vi "CameraControl.vi"() -> ()   [LabVIEW 2013]
uses:
  QImaging_Basic/Controls/Parameter.ctl
panel:
  out "abort err":errorcluster
  in  "Abort":bool
  in  "Trig":bool
  out "Intensity Graph":u16[][](graph)
  out "CCD Height":u32=1 min=1 max=4 step=1
  out "CCD Width":u32=1 min=1 max=4 step=1
  in  "Binning":u32=1 min=1 max=4 step=1
  out "Open Cam Error":i32
  out "LibCam Error":u32
  out "LibOpen error":i32
  in  "Stop Camera":bool
  in  "Start Camera":bool
  in  "Exposure Time":u32
  out "ParamVal":u32[](array[numeric])
  out "Camera Id":u32
  out "error out":errorcluster
  in  "error in (no error)":errorcluster
  in  "Stop":bool
  # "Hardware"
  # "Freerun"
  # "Image Width"
  # "Image Height"
  # "Image Size"
  # "CCD Type"
  # "CCD Width"
  # "CCD Height"
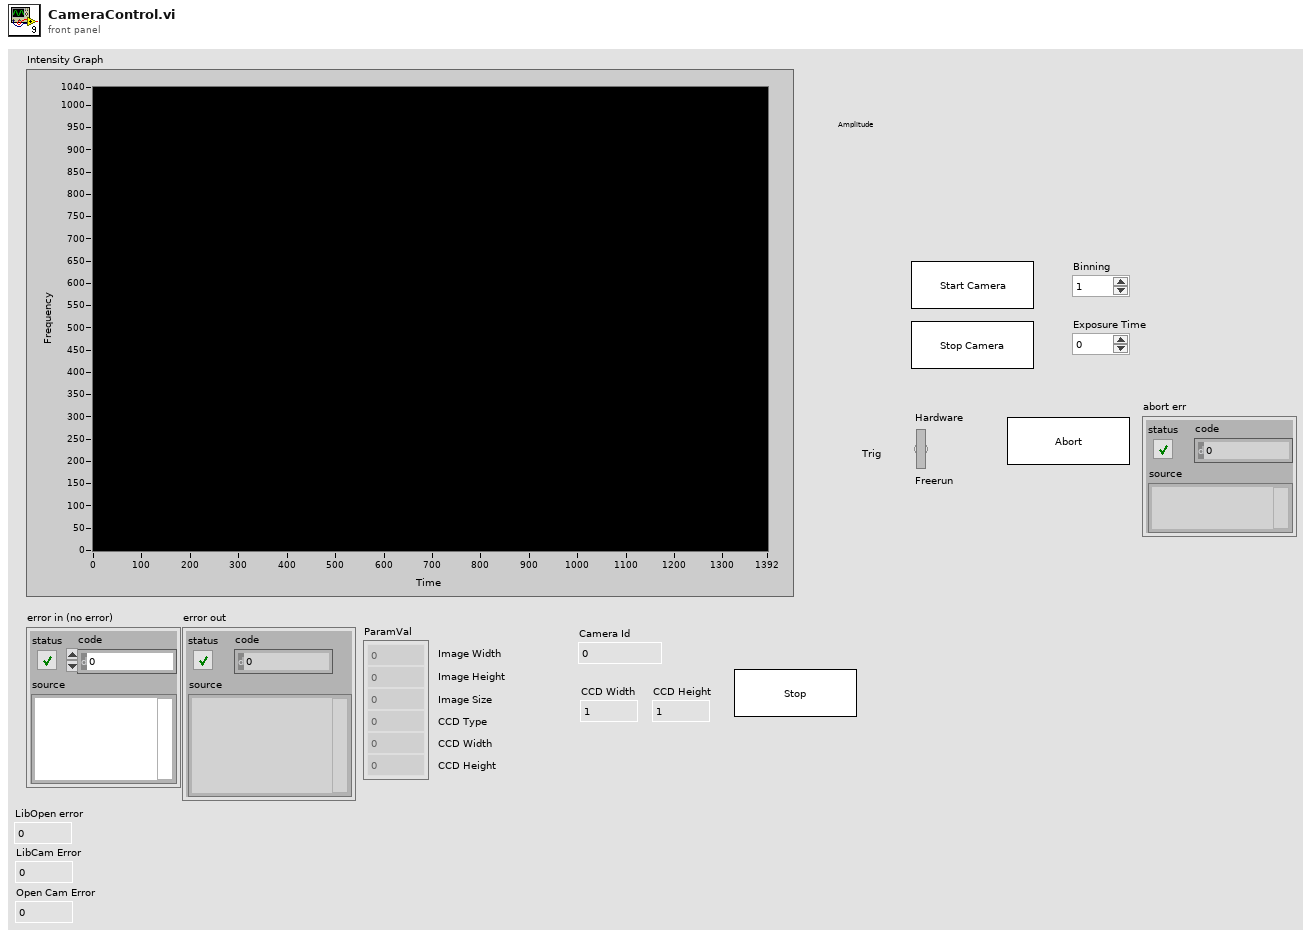
[diagram p1: front panel]
types:
  T1 = typedef "Parameter.ctl" = enum32{"Gain ", "Offset", "Exposure", "Binning", "HzBinning", "VtBinning", "Readout speed", "Trigger Type", "Color Wheel", "Cooler Active", "Exposure red", "Exposure blue", "Image format", "ROI X", "ROI Y", "ROI Width", "ROI Height"}
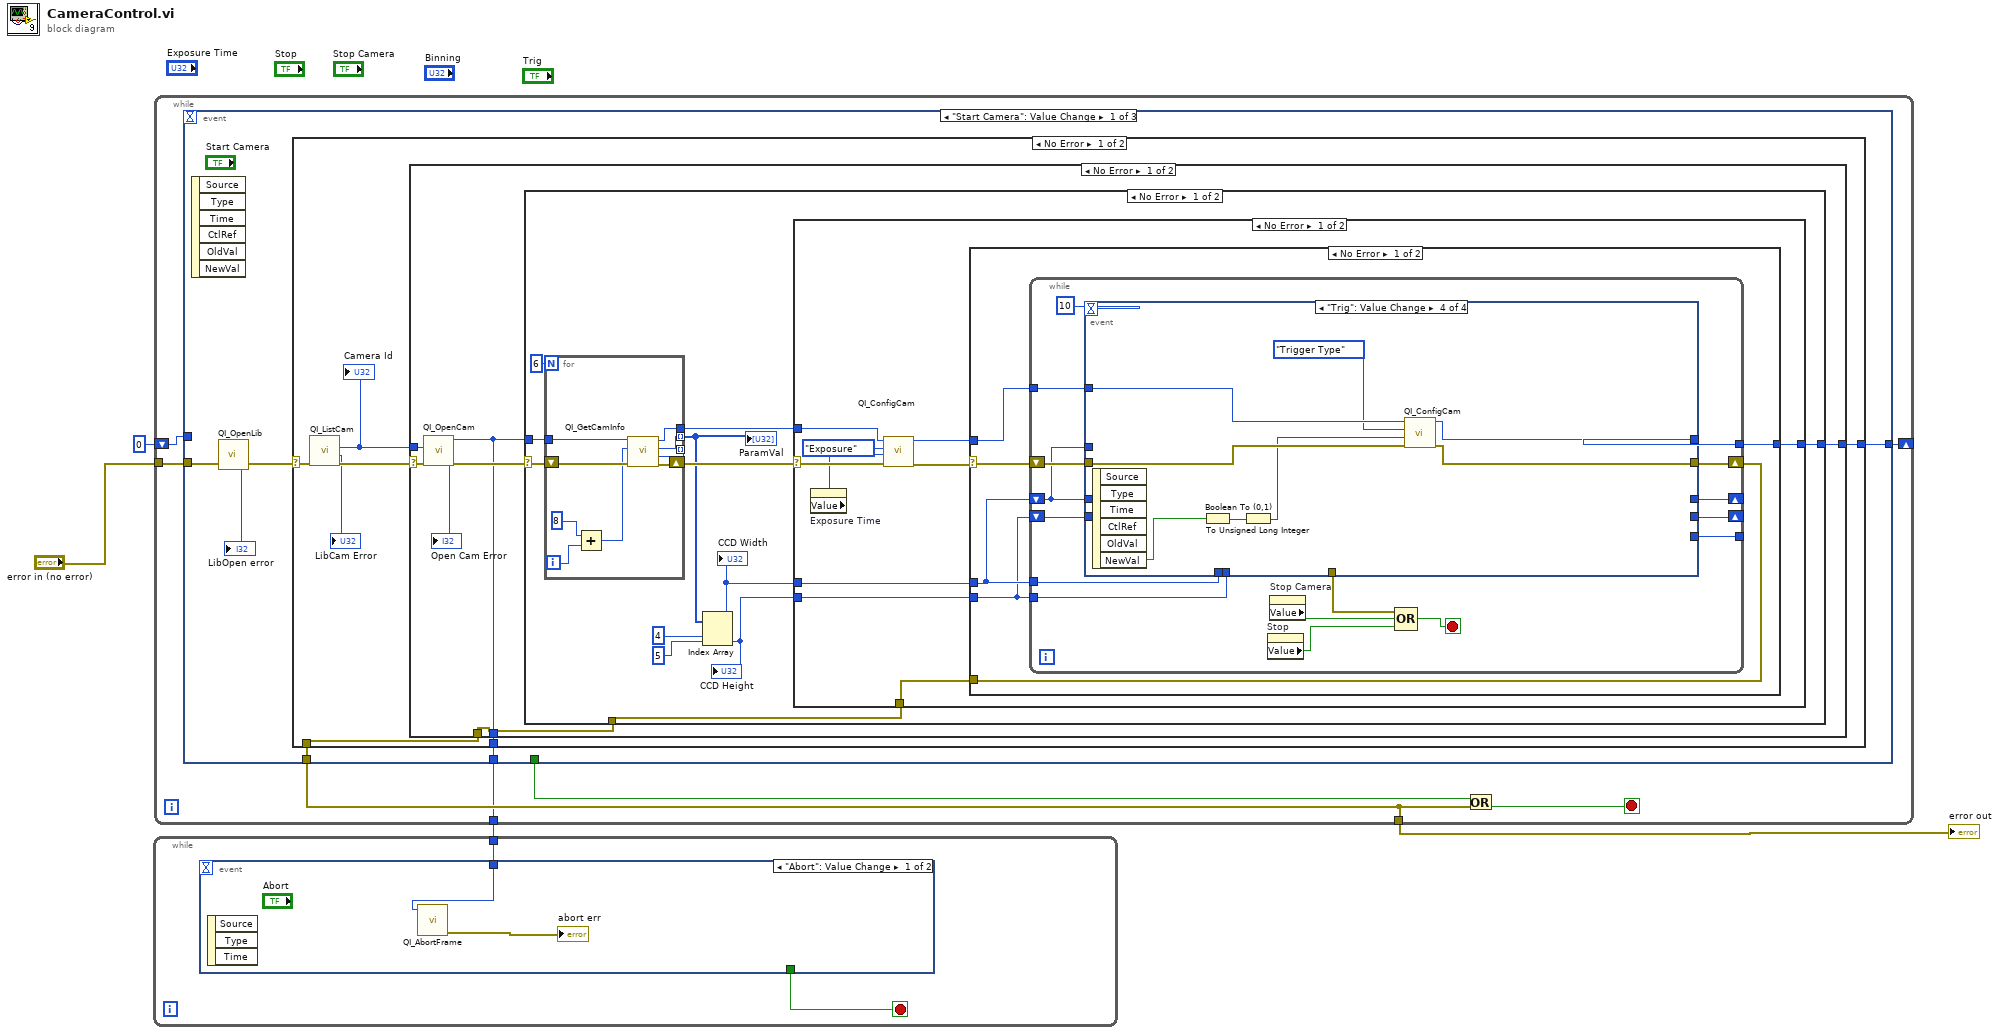
[diagram p0: block diagram]
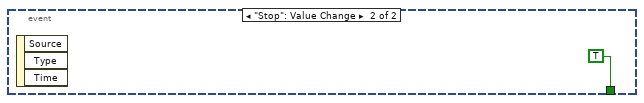
[diagram p2: hidden frame]
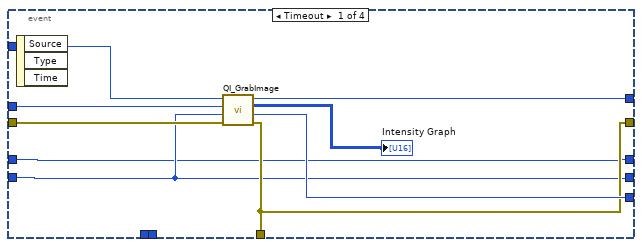
[diagram p3: hidden frame]
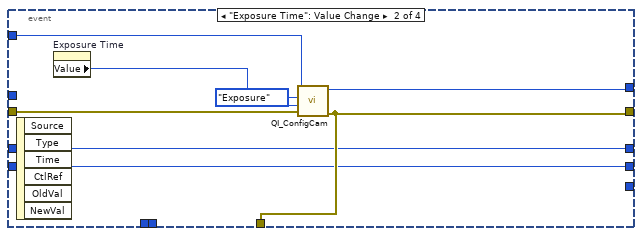
[diagram p4: hidden frame]
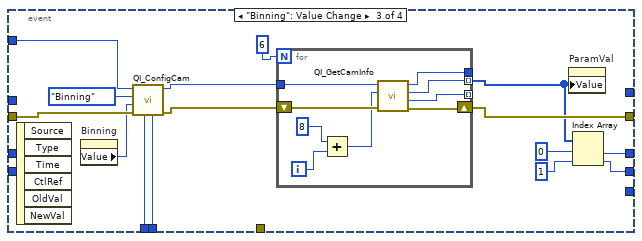
[diagram p5: hidden frame]
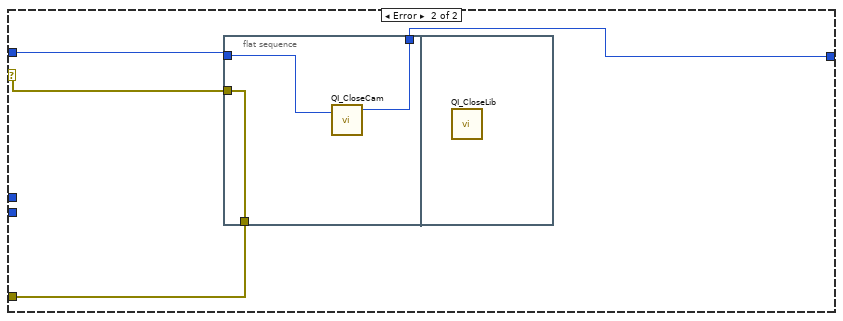
[diagram p6: hidden frame]
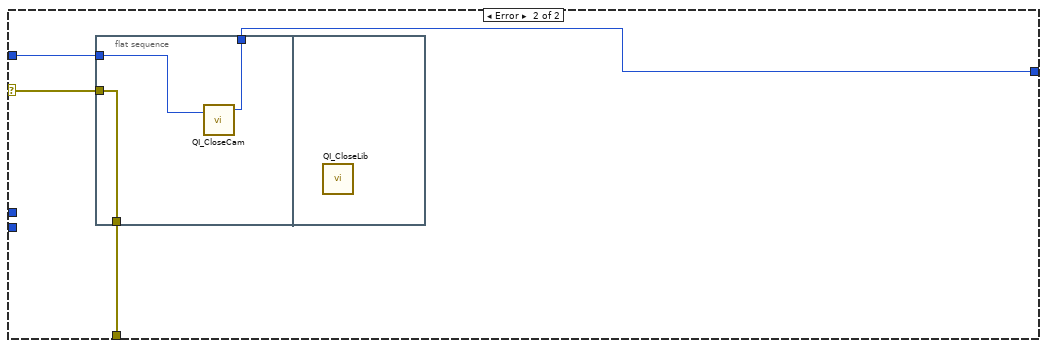
[diagram p7: hidden frame]
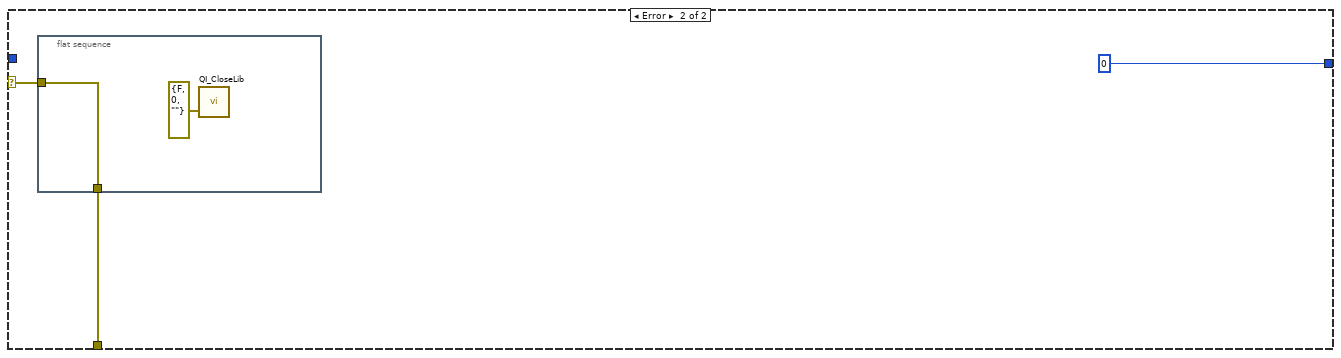
[diagram p8: hidden frame]
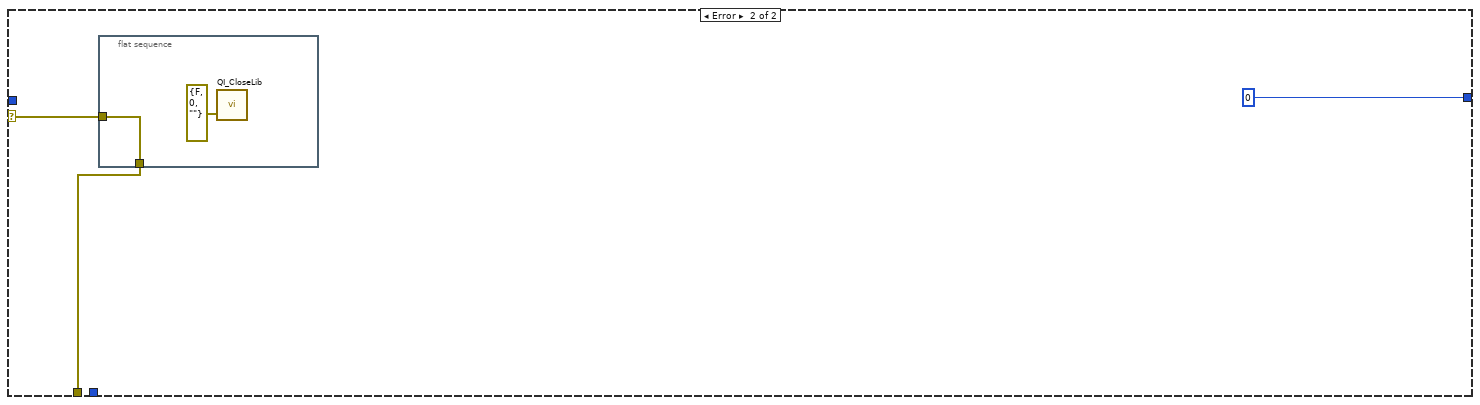
[diagram p9: hidden frame]
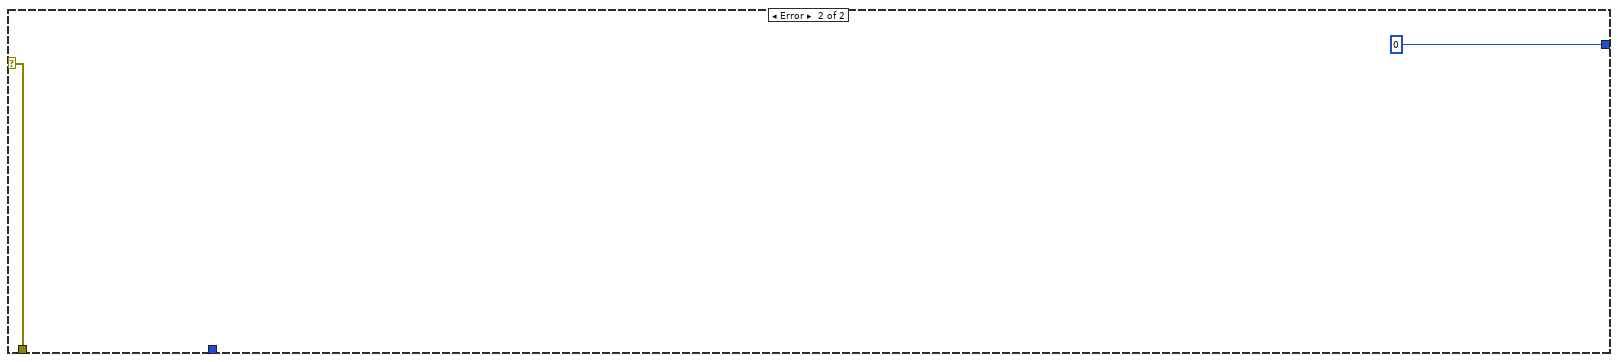
[diagram p10: hidden frame]
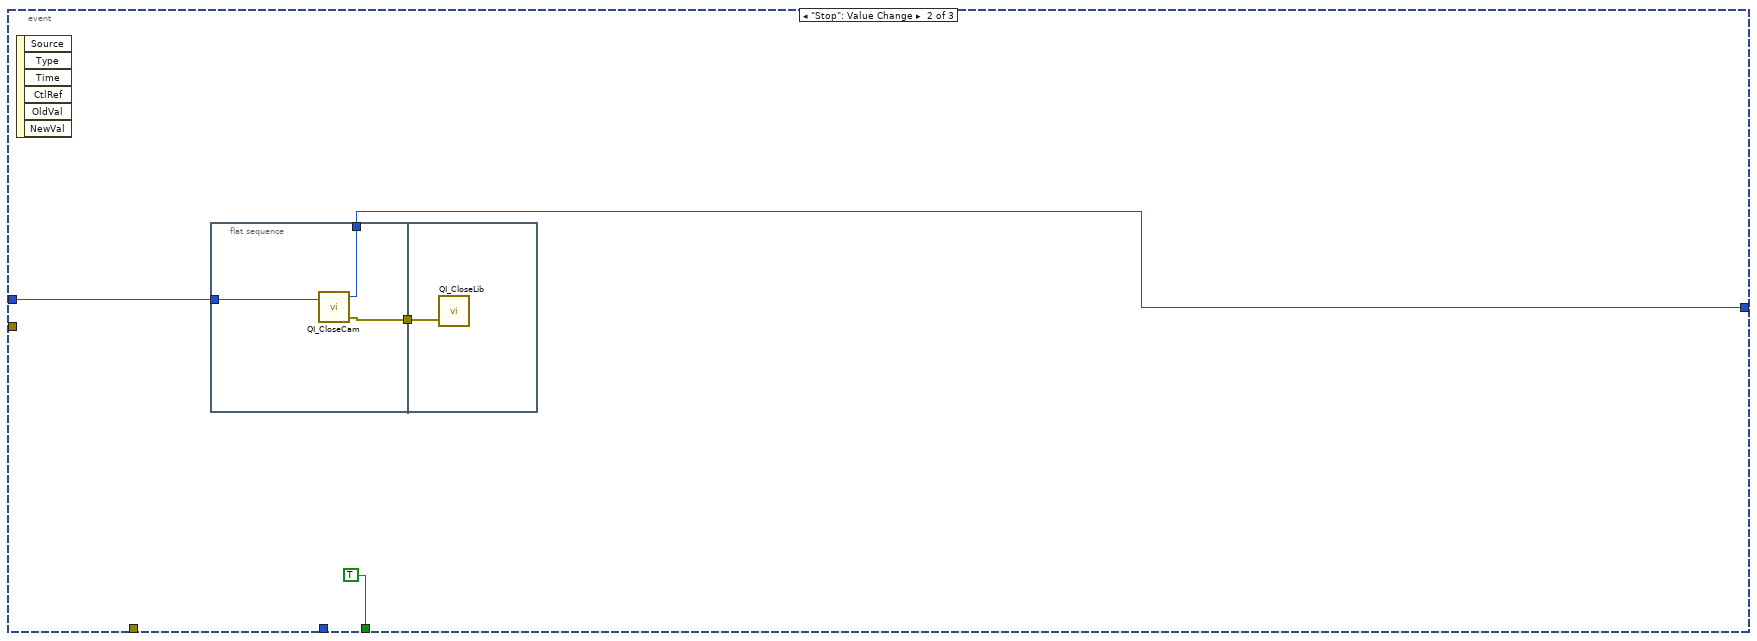
[diagram p11: hidden frame]
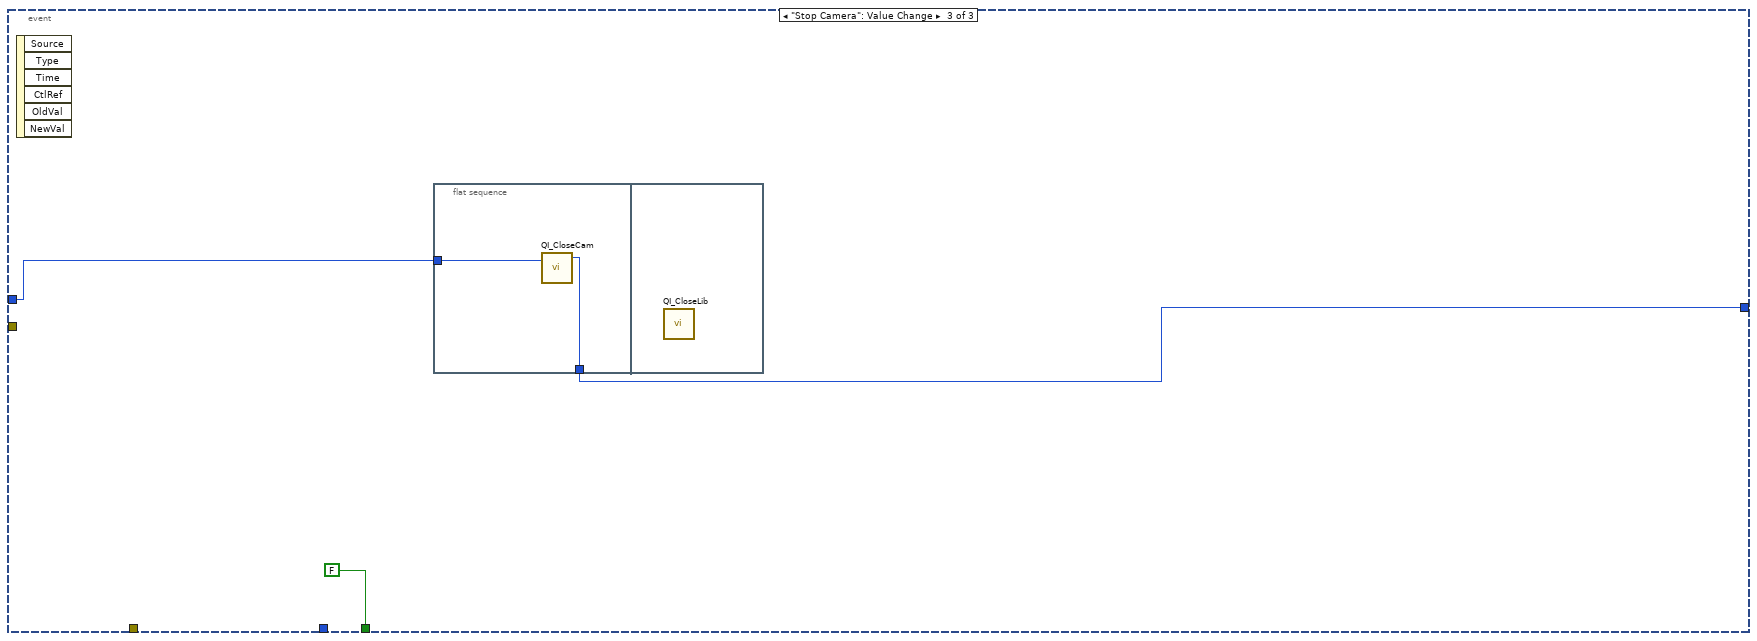
[diagram p12: hidden frame]
diagram:
  n1 = while {
    tunnel: "error in (no error)" -> [w11]
    shift-right: [w9] -> _
    shift-left: u32 0 ("Camera Handle") -> [w8]
    tunnel: [w7] -> w2
    tunnel: [w5] -> w1
    stop <- w6 stop-if-true
    n2 = event shown="[0] \"Start Camera\": Value Change" {
      selector: _ -> [_ _ _]
      dyn-events: _ -> [_ _ _]
      timeout: _ -> [_ _ _]
      tunnel: w11 -> [w17 _ _]
      tunnel: [w15 _ _] -> w7
      tunnel: [_ TRUE FALSE] -> w10
      tunnel: [w14 w160 w168] -> w9
      tunnel: w8 -> [_ w162 w170]
      tunnel: [w12 _ _] -> w5
      event "Start Camera": Value Change {
        n3 = event-data() -> ()  [unwired: 1 in, 6 out]
        n4 = call "QI_OpenLib.vi"("error in (no error)"=w17) -> ("error out"=w16:errorcluster, "LibOpen error"=→"LibOpen error":i32)  [unwired: 1 in]
        n5 = case shown="No Error" w16 {
          selector: w16 -> [w24 w159]
          tunnel: [w21 w159] -> w15
          tunnel: [w20 u32 0 ("Camera Handle")] -> w14
          tunnel: [w18 _] -> w12
          frame No Error {
            n6 = call "QI_ListCam.vi"("error in (no error)"=w24) -> ("error out"=w23:errorcluster, "LibCam Error"=→"LibCam Error":u32, "cameraId"=w22:u32)  [unwired: 8 in]
            "Camera Id" <- w22
            n7 = case shown="No Error" w23 {
              selector: w23 -> [w31 w155]
              tunnel: w22 -> [w30 _]
              tunnel: [w28 w154] -> w21
              tunnel: [w27 u32 0 ("Camera Handle")] -> w20
              tunnel: [w25 _] -> w18
              frame No Error {
                n8 = call "QI_OpenCam.vi"("error in (no error)"=w31, "Camera ID"=w30) -> ("error out"=w29:errorcluster, "Open Cam Error"=→"Open Cam Error":i32, "Camera Handle"=w25:u32)  [unwired: 7 in]
                n9 = case shown="No Error" w29 {
                  selector: w29 -> [w43 w150]
                  tunnel: w25 -> [w42 _]
                  tunnel: [w38 w149] -> w28
                  tunnel: [w37 u32 0 ("Camera Handle")] -> w27
                  frame No Error {
                    n10 = for {
                      N: 6 -> [_]
                      tunnel: w42 -> [w146]
                      shift-right: [w142] -> w40
                      shift-left: w43 -> [w147]
                      tunnel: [w141] -> w39
                      tunnel: [w140] -> w36 mode=indexing
                      tunnel: [w139] -> _ mode=indexing
                      i -> [w145]
                      n11 = Add(x=u32 8, y=w145) -> (x+y=w143:u32)
                      n12 = call "QI_GetCamInfo.vi"("error in (no error)"=w147, "paramKey"=w143, "Camera Handle"=w146) -> ("error out"=w142:errorcluster, "CamInfo err"=w139:i32, "paramVal"=w140:u32, "Camera Handle"=w141:u32)  [unwired: 5 in]
                    }
                    "ParamVal" <- w36
                    n13 = Index Array(array=w36, index #1=4 ("index"), index #2=5 ("index")) -> (element #1=w33:u32, element #2=w32:u32)
                    "CCD Width" <- w33
                    "CCD Height" <- w32
                    n14 = case shown="No Error" w40 {
                      selector: w40 -> [w53 w135]
                      tunnel: w39 -> [w52 w133]
                      tunnel: [w48 w134] -> w38
                      tunnel: [w47 w132] -> w37
                      tunnel: w33 -> [w45 _]
                      tunnel: w32 -> [w44 _]
                      frame No Error {
                        n15 = property on="Exposure Time" class="DigNum (strict)"() -> ("Value"=w51:u32)  [unwired: 2 in, 2 out]
                        n16 = call "QI_ConfigCam.vi"("error in (no error)"=w53, "paramVal"=w51, "Parameter"=Parameter."Exposure", "Camera Handle"=w52) -> ("error out"=w49:errorcluster, "Camera Handle"=w50:u32)  [unwired: 5 in, 1 out]
                        n17 = case shown="No Error" w49 {
                          selector: w49 -> [w58 w127]
                          tunnel: w50 -> [w59 w128]
                          tunnel: w45 -> [w55 _]
                          tunnel: w44 -> [w54 _]
                          tunnel: [w56 w126] -> w48
                          tunnel: [w57 w125] -> w47
                          frame No Error {
                            n18 = while {
                              tunnel: w59 -> [w75]
                              tunnel: [w69] -> _
                              tunnel: [w67] -> w57
                              shift-right: [w66] -> w56
                              shift-left: w58 -> [w74]
                              shift-right: [w65] -> _
                              shift-left: w55 -> [w62]
                              shift-right: [w64] -> _
                              shift-left: w54 -> [w63]
                              tunnel: w55 -> [w61]
                              tunnel: w54 -> [w60]
                              stop <- w71 stop-if-true
                              n19 = event shown="[3] \"Trig\": Value Change" {
                                selector: _ -> [_ _ _ _]
                                dyn-events: _ -> [_ _ _ _]
                                timeout: 10 -> [_ _ _ _]
                                tunnel: w75 -> [w84 w92 w107 w124]
                                tunnel: w74 -> [w83 w89 w105 w121]
                                tunnel: w62 -> [w82 _ _ _]
                                tunnel: [w79 w88 _ _] -> w73
                                tunnel: [w81 w91 _ w123] -> w67
                                tunnel: [w80 _ _ _] -> w69
                                tunnel: [w79 w88 w104 w122] -> w66
                                tunnel: [w77 w87 w100 _] -> w65
                                tunnel: [w78 w86 w99 _] -> w64
                                tunnel: w63 -> [w78 w86 _ _]
                                tunnel: w62 -> [w77 w87 _ _]
                                tunnel: w61 -> [_ _ w94 _]
                                tunnel: w60 -> [_ _ w93 _]
                                event Timeout {
                                n20 = event-data() -> ()  [unwired: 1 in, 3 out]
                                n21 = call "QI_GrabImage.vi"("error in (no error)"=w83, "Image Width"=w78, "Image Height"=w82, "Camera Handle"=w84) -> ("error out"=w79:errorcluster, "GrabImage err"=w80:u32, "data"=→"Intensity Graph":u16[][], "Camera Handle"=w81:u32)  [unwired: 4 in]
                                }
                                event "Exposure Time": Value Change {
                                n22 = event-data() -> ()  [unwired: 1 in, 6 out]
                                n23 = property on="Exposure Time" class="DigNum (strict)"() -> ("Value"=w90:u32)  [unwired: 2 in, 2 out]
                                n24 = call "QI_ConfigCam.vi"("error in (no error)"=w89, "paramVal"=w90, "Parameter"=Parameter."Exposure", "Camera Handle"=w92) -> ("error out"=w88:errorcluster, "Camera Handle"=w91:u32)  [unwired: 5 in, 1 out]
                                }
                                event "Binning": Value Change {
                                n25 = event-data() -> ()  [unwired: 1 in, 6 out]
                                n26 = property on="Binning" class="DigNum (strict)"() -> ("Value"=w97:u32)  [unwired: 2 in, 2 out]
                                n27 = call "QI_ConfigCam.vi"("CCD Height"=w93, "CCD Width"=w94, "error in (no error)"=w105, "paramVal"=w97, "Parameter"=Parameter."Binning", "Camera Handle"=w107) -> ("error out"=w96:errorcluster, "Camera Handle"=w98:u32)  [unwired: 3 in, 1 out]
                                n28 = for {
                                N: 6 -> [_]
                                shift-right: [w112] -> w104
                                shift-left: w96 -> [w116]
                                tunnel: [w111] -> _
                                tunnel: [w110] -> w103 mode=indexing
                                tunnel: [w109] -> _ mode=indexing
                                tunnel: w98 -> [w108]
                                i -> [w115]
                                n29 = Add(x=u32 8, y=w115) -> (x+y=w113:u32)
                                n30 = call "QI_GetCamInfo.vi"("error in (no error)"=w116, "paramKey"=w113, "Camera Handle"=w108) -> ("error out"=w112:errorcluster, "CamInfo err"=w109:i32, "paramVal"=w110:u32, "Camera Handle"=w111:u32)  [unwired: 5 in]
                                }
                                n31 = property on="ParamVal" class="Arr (strict)"("Value"=w103) -> ()  [unwired: 2 in, 2 out]
                                n32 = Index Array(array=w103, index #1=0 ("index"), index #2=1 ("index")) -> (element #1=w100:u32, element #2=w99:u32)
                                }
                                event "Trig": Value Change {
                                n33 = event-data() -> ("NewVal"=w119:bool)  [unwired: 1 in, 5 out]
                                n34 = Boolean To (0,1)(Boolean=w119) -> (0, 1=w118:i16)
                                n35 = To Unsigned Long Integer(number=w118) -> (unsigned 32bit integer=w117:u32)
                                n36 = call "QI_ConfigCam.vi"("error in (no error)"=w121, "paramVal"=w117, "Parameter"=Parameter."Trigger Type", "Camera Handle"=w124) -> ("error out"=w122:errorcluster, "Camera Handle"=w123:u32)  [unwired: 5 in, 1 out]
                                }
                              }
                              n37 = property on="Stop" class="Bool (strict)"() -> ("Value"=w68:bool)  [unwired: 2 in, 2 out]
                              n38 = property on="Stop Camera" class="Bool (strict)"() -> ("Value"=w72:bool)  [unwired: 2 in, 2 out]
                              n39 = Compound Arithmetic op=OR(w73, w72, w68) -> (w71:bool)
                            }
                          }
                          frame Error {
                            n40 = flat-sequence {
                              tunnel: w127 -> [w130]
                              tunnel: [w130] -> w126
                              tunnel: w128 -> [w131]
                              tunnel: [w129] -> w125
                              frame #0 {
                                n41 = call "QI_CloseCam.vi"("Camera Handle"=w131) -> ("Camera Handle"=w129:u32)  [unwired: 1 in, 2 out]
                              }
                              frame #1 {
                                n42 = call "QI_CloseLib.vi"() -> ()  [unwired: 2 in, 2 out]
                              }
                            }
                          }
                        }
                      }
                      frame Error {
                        n43 = flat-sequence {
                          tunnel: w135 -> [w137]
                          tunnel: [w137] -> w134
                          tunnel: w133 -> [w138]
                          tunnel: [w136] -> w132
                          frame #0 {
                            n44 = call "QI_CloseCam.vi"("Camera Handle"=w138) -> ("Camera Handle"=w136:u32)  [unwired: 1 in, 2 out]
                          }
                          frame #1 {
                            n45 = call "QI_CloseLib.vi"() -> ()  [unwired: 2 in, 2 out]
                          }
                        }
                      }
                    }
                  }
                  frame Error {
                    n46 = flat-sequence {
                      tunnel: w150 -> [w152]
                      tunnel: [w152] -> w149
                      frame #0 {
                        n47 = call "QI_CloseLib.vi"("error in (no error)"=errorcluster {"status"=FALSE, "code"=0, "source"=""}) -> ()  [unwired: 1 in, 2 out]
                      }
                    }
                  }
                }
              }
              frame Error {
                n48 = flat-sequence {
                  tunnel: w155 -> [w157]
                  tunnel: [w157] -> w154
                  frame #0 {
                    n49 = call "QI_CloseLib.vi"("error in (no error)"=errorcluster {"status"=FALSE, "code"=0, "source"=""}) -> ()  [unwired: 1 in, 2 out]
                  }
                }
              }
            }
          }
          frame Error {
          }
        }
      }
      event "Stop": Value Change {
        n50 = event-data() -> ()  [unwired: 1 in, 6 out]
        n51 = flat-sequence {
          tunnel: w162 -> [w166]
          tunnel: [w165] -> w161
          tunnel: [w164] -> w160
          tunnel: w161 -> [w167]
          frame #0 {
            n52 = call "QI_CloseCam.vi"("Camera Handle"=w166) -> ("Camera Handle"=w164:u32, "error out"=w165:errorcluster)  [unwired: 1 in, 1 out]
          }
          frame #1 {
            n53 = call "QI_CloseLib.vi"("error in (no error)"=w167) -> ()  [unwired: 1 in, 2 out]
          }
        }
      }
      event "Stop Camera": Value Change {
        n54 = event-data() -> ()  [unwired: 1 in, 6 out]
        n55 = flat-sequence {
          tunnel: w170 -> [w172]
          tunnel: [w171] -> w168
          frame #0 {
            n56 = call "QI_CloseCam.vi"("Camera Handle"=w172) -> ("Camera Handle"=w171:u32)  [unwired: 1 in, 2 out]
          }
          frame #1 {
            n57 = call "QI_CloseLib.vi"() -> ()  [unwired: 2 in, 2 out]
          }
        }
      }
    }
    n58 = Or(x=w10, y=w7) -> (x .or. y?=w6:bool)
  }
  "error out" <- w2
  n59 = while {
    tunnel: w1 -> [w174]
    stop <- w173 stop-if-true
    n60 = event shown="[0] \"Abort\": Value Change" {
      selector: _ -> [_ _]
      dyn-events: _ -> [_ _]
      timeout: _ -> [_ _]
      tunnel: w174 -> [w176 _]
      tunnel: [_ TRUE] -> w173
      event "Abort": Value Change {
        n61 = event-data() -> ()  [unwired: 1 in, 3 out]
        n62 = call "QI_AbortFrame.vi"("Camera Handle"=w176) -> ("error out"=→"abort err":errorcluster)  [unwired: 9 in, 1 out]
      }
      event "Stop": Value Change {
        n63 = event-data() -> ()  [unwired: 1 in, 3 out]
      }
    }
  }
